vi "open_itxFolder_to_labview.vi"(8 "error in (no error)":errorcluster, 10 "experiment folder (containing itx)":path) -> (0 "error out":errorcluster, 3 "Whole folder ITX data":dbl[][][](array[numeric]))   [LabVIEW 2016]
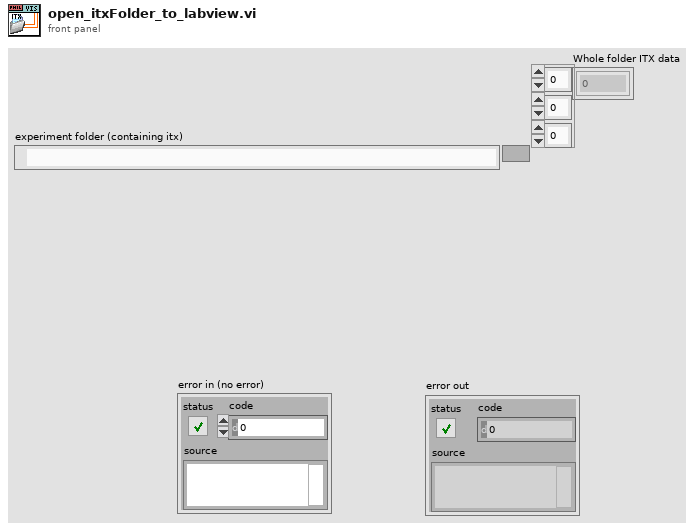
[diagram p1: front panel]
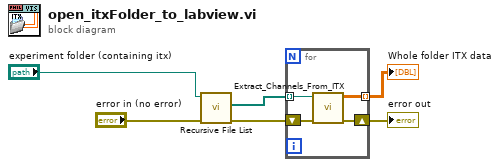
[diagram p0: block diagram]
diagram:
  n1 = call <vilib>:"Recursive File List.vi"("error in (no error)"="error in (no error)", "Folder Path"="experiment folder (containing itx)") -> ("error out"=w1:errorcluster, "All Files in Dir"=w2:path[])  [unwired: 5 in, 3 out]
  n2 = for {
    tunnel: w2 -> [w10] mode=indexing
    shift-right: [w8] -> w4
    shift-left: w1 -> [w9]
    tunnel: [w7] -> w3 mode=indexing
    n3 = call "Extract_Channels_From_ITX.vi"("error in"=w9, "itx file, N 1d channels"=w10) -> ("error out"=w8:errorcluster, "Arr of 1D channels"=w7:dbl[][])  [unwired: 5 in, 3 out]
  }
  "error out" <- w4
  "Whole folder ITX data" <- w3
